vi "GetFlowData (SubVI).vi"(7 "error in (no error)":errorcluster, 9 "Node":u8, 10 "VISA Refnum in":refnum<visa-resource-name>) -> (0 "error out":errorcluster, 2 "Flow Data":T1)   [LabVIEW 2015]
uses:
  TypeDefs/FlowData.ctl
  <instrlib>/Bronkhorst FLOW-BUS/Public/Data/Setpoint/Read Setpoint (Direct).vi
  <instrlib>/Bronkhorst FLOW-BUS/Public/Data/Setpoint/Read Setpoint (Percentage).vi
  <instrlib>/Bronkhorst FLOW-BUS/Public/Data/Measure/Read Measure (Direct).vi
  <instrlib>/Bronkhorst FLOW-BUS/Public/Data/Measure/Read Measure (Percentage).vi
  FlowFilmVariable.vi
  <instrlib>/Bronkhorst FLOW-BUS/Bronkhorst FLOW-BUS.lvlib
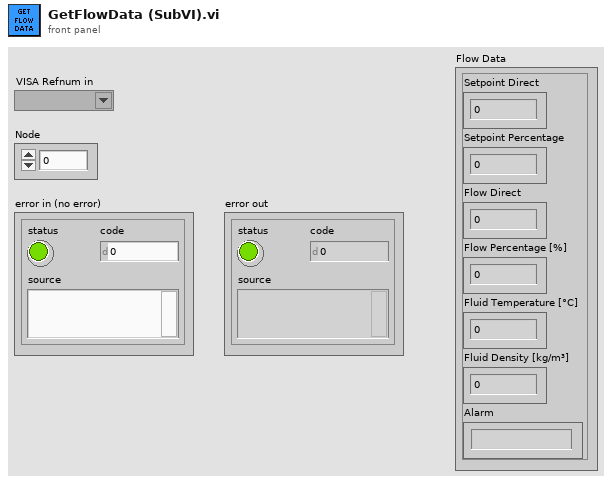
[diagram p1: front panel]
types:
  T1 = typedef "FlowData.ctl" = cluster{"Setpoint Direct":sgl, "Setpoint Percentage":dbl, "Flow Direct":sgl, "Flow Percentage [%]":dbl, "Fluid Temperature [°C]":sgl, "Fluid Density [kg/m³]":sgl, "Alarm":string}
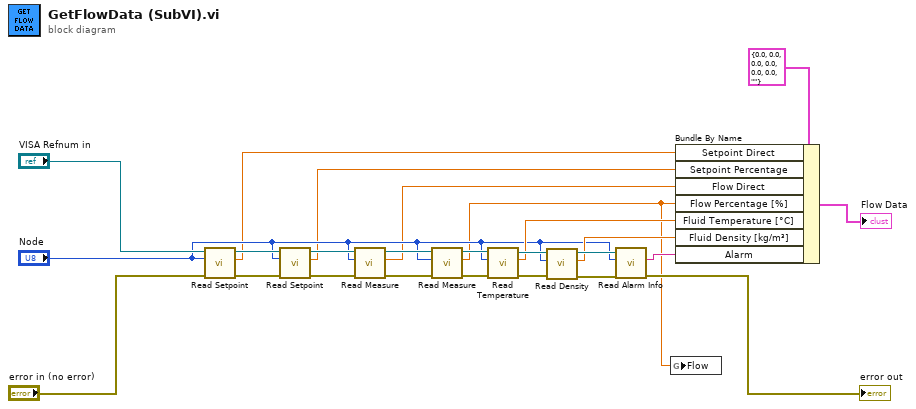
[diagram p0: block diagram]
diagram:
  n1 = call-poly <instrlib>:"Read Setpoint.vi"("error in (no error)"="error in (no error)", "Node (3)"="Node", "VISA resource name"="VISA Refnum in") -> ("error out"=w8:errorcluster, "Setpoint Direct"=w3:sgl, "VISA resource name out"=w10:refnum<visa-resource-name>)  [unwired: 6 in]
  n2 = call-poly <instrlib>:"Read Setpoint.vi"("error in (no error)"=w8, "Node (3)"="Node", "VISA resource name"=w10) -> ("error out"=w7:errorcluster, "Setpoint Percentage"=w4:dbl, "VISA resource name out"=w11:refnum<visa-resource-name>)  [unwired: 6 in]
  n3 = call-poly <instrlib>:"Read Measure.vi"("error in (no error)"=w7, "Node (3)"="Node", "VISA resource name"=w11) -> ("error out"=w23:errorcluster, "Measure Direct"=w2:sgl, "VISA resource name out"=w24:refnum<visa-resource-name>)  [unwired: 6 in]
  n4 = call-poly <instrlib>:"Read Measure.vi"("error in (no error)"=w23, "Node (3)"="Node", "VISA resource name"=w24) -> ("error out"=w20:errorcluster, "Measure Percentage"=w1:dbl, "VISA resource name out"=w21:refnum<visa-resource-name>)  [unwired: 6 in]
  n5 = call <instrlib>:"Read Temperature.vi"("error in (no error)"=w20, "Node (3)"="Node", "VISA resource name"=w21) -> ("error out"=w19:errorcluster, "Temperature (deg C)"=w15:sgl, "VISA resource name out"=w17:refnum<visa-resource-name>)  [unwired: 6 in]
  n6 = call <instrlib>:"Read Density.vi"("error in (no error)"=w19, "Node (3)"="Node", "VISA resource name"=w17) -> ("error out"=w18:errorcluster, "Density (kg/m3)"=w14:sgl, "VISA resource name out"=w16:refnum<visa-resource-name>)  [unwired: 6 in]
  n7 = call <instrlib>:"Read Alarm Info.vi"("error in (no error)"=w18, "Node (3)"="Node", "VISA resource name"=w16) -> ("error out"=→"error out":errorcluster, "Alarm Message"=w13:string)  [unwired: 6 in, 1 out]
  n8 = global write "FlowFilmVariable.vi" "Flow"(w1) -> ()
  n9 = Bundle By Name(cluster=T1 {"Setpoint Direct"=0.0, "Setpoint Percentage"=0.0, "Flow Direct"=0.0, "Flow Percentage [%]"=0.0, "Fluid Temperature [°C]"=0.0, "Fluid Density [kg/m³]"=0.0, "Alarm"=""} ("Sensor Data"), "Setpoint Direct"=w3, "Setpoint Percentage"=w4, "Flow Direct"=w2, "Flow Percentage [%]"=w1, "Fluid Temperature [°C]"=w15, "Fluid Density [kg/m³]"=w14, "Alarm"=w13) -> (→"Flow Data":T1)
